vi "Lian_Lab09_II.vi"() -> ()   [LabVIEW 2020]
uses:
  <vilib>/DAQmx/read.llb/DAQmx Read (Analog Wfm 1Chan NSamp).vi
  <vilib>/DAQmx/create/channels.llb/DAQmx Create Channel (AI-Voltage-Basic).vi
  <vilib>/DAQmx/configure/timing.llb/DAQmx Timing (Sample Clock).vi
  <vilib>/measure/macond.llb/IIR Filter for 1 Chan.vi
  <vilib>/measure/maspectr.llb/FFT Spectrum (Mag-Phase) for 1 Chan.vi
  <vilib>/DAQmx/miscellaneous.llb/DAQmx Fill In Error Info.vi
  <vilib>/measure/NI_MAPro.lvlib
  <resource>/objmgr/daqmx.rc
panel:
  out "# Elements \nin Queue":i32
  out "Consumer\nIterations":i32
  out "Producer \nIterations":i32
  out "Actual Rate":dbl
  in  "?":enum32{"Channel", "Sampling", "Filter"}(tab)
  in  "Physical Channels":tag="myDAQ1/ai0"
  in  "Maximum Voltage":dbl=10.0 format="%0.2f"
  in  "Minimum Voltage":dbl=-10.0 format="%0.2f"
  in  "Input Terminal Config.":i32(ring)=10106 items=["Default"=-1, "RSE"=10083, "NRSE"=10078, "Differential"=10106, "Pseudodifferential"=12529]
  in  "Loop Multiple (ms)":u32=1000
  in  "# Samples  per Channel":i32=40000
  in  "Requested Rate":dbl=80000.0 format="%0.2f"
  in  "Samples per Channel":i32=800000
  in  "IIR Specifications":T1={"Topology"=enum."Butterworth", "Type"=enum."Highpass", "Order"=3, "Lower Fc"=100.0, "Upper Fc"=200.0, "PB Ripple"=1.0, "SB Attenuation"=60.0} {"PB Ripple" format="%0.2f"; "SB Attenuation" format="%0.2f"; "Lower Fc" format="%0.2p"; "Upper Fc" format="%0.2p"}
  in  "?":bool
  out "Voltage":waveform(dbl)(graph)
  out "FFT":cluster{"f0":dbl, "df":dbl, "magnitude":dbl[]}(graph)
  # "Settings"
  # "Info"
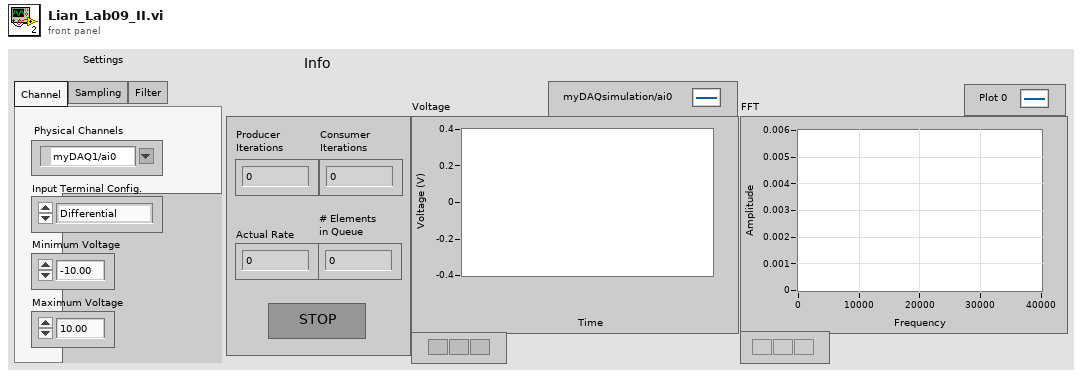
[diagram p1: front panel]
types:
  T1 = cluster{"Topology":enum16{"Off", "Butterworth", "Chebyshev", "Inverse Chebyshev", "Elliptic", "Bessel"}, "Type":enum16{"Lowpass", "Highpass", "Bandpass", "Bandstop"}, "Order":i32, "Lower Fc":dbl, "Upper Fc":dbl, "PB Ripple":dbl, "SB Attenuation":dbl}
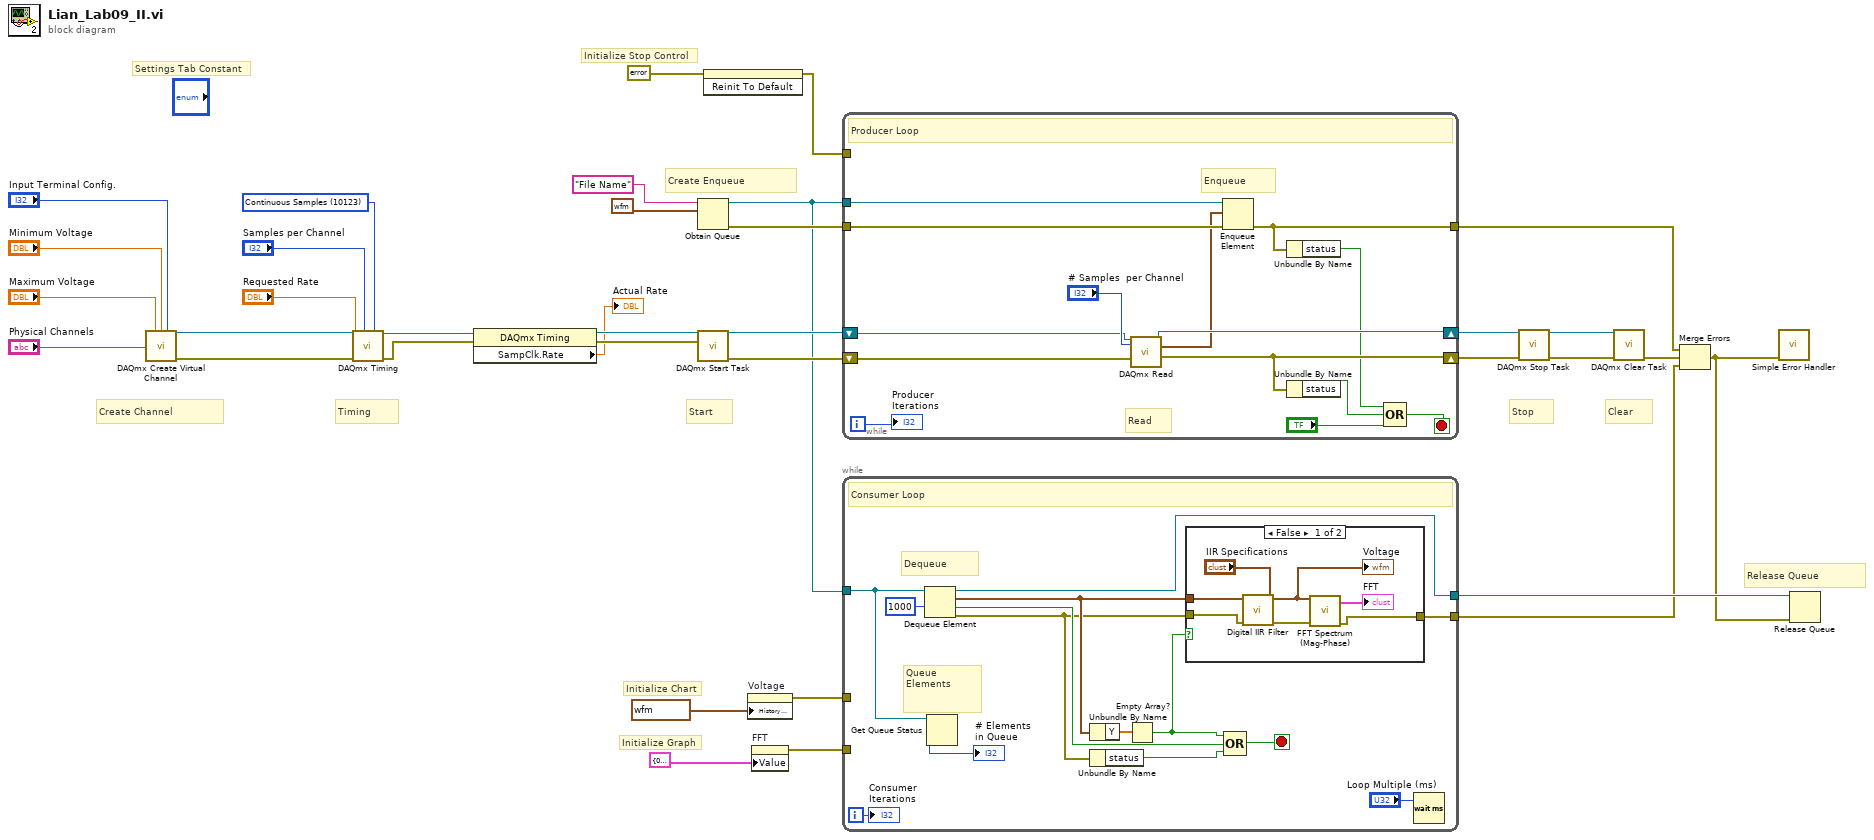
[diagram p0: block diagram]
diagram:
  w21 = 10123 items=["Finite Samples"=10178, "Continuous Samples"=10123, "Hardware Timed Single Point"=12522] ("sample mode")
  # "Initialize Stop Control"
  # "Release Queue"
  # "Create Enqueue"
  # "Clear"
  # "Stop"
  # "Start"
  # "Timing"
  # "Create Channel"
  # "Settings Tab Constant"
  # "Initialize Graph"
  # "Initialize Chart"
  n1 = call-poly <vilib>:"DAQmx Create Virtual Channel.vi"("maximum value"="Maximum Voltage", "minimum value"="Minimum Voltage", "input terminal configuration"="Input Terminal Config.", "physical channels"="Physical Channels") -> ("task out"=w26:refnum<k21>, "error out"=w30:errorcluster)  [unwired: 10 in]
  n2 = call-poly <vilib>:"DAQmx Timing.vi"("task/channels in"=w26, "sample mode"=w21, "samples per channel"="Samples per Channel", "rate"="Requested Rate", "error in"=w30) -> ("task out"=w20:refnum<k21>, "error out"=w18:errorcluster)  [unwired: 9 in]
  n3 = property class="DAQmx Timing"(reference=w20, error in=w18) -> (reference out=w19:refnum<k21>, error out=w17:errorcluster, "SampClk.Rate"=→"Actual Rate":dbl)
  n4 = Obtain Queue(name (unnamed)="File Name", element data type=waveform(dbl) {"t0"=timestamp(0 s since 1904-01-01), "dt"=0.0, "Y"=[]} ("Waveform")) -> (queue out=w12:refnum<queue>, error out=w15:errorcluster)  [unwired: 3 in, 1 out]
  n5 = call <vilib>:"DAQmx Start Task.vi"("task/channels in"=w19, "error in"=w17) -> ("task out"=w25:refnum<k21>, "error out"=w29:errorcluster)  [unwired: 12 in]
  n6 = invoke class="Bool (strict)" method="Reinit To Default"(error in=errorcluster {"status"=FALSE, "code"=0, "source"=""} ("error in (no error)")) -> (error out=w4:errorcluster)  [unwired: 2 in, 2 out]
  n7 = property on="Voltage" class="WFChart (strict)"("History Data"=waveform(dbl)[] [{"t0"=timestamp(0 s since 1904-01-01), "dt"=0.0, "Y"=[]}]) -> (error out=w9:errorcluster)  [unwired: 2 in, 1 out]
  n8 = property on="FFT" class="WFGraph (strict)"("Value"=cluster{"f0":dbl, "df":dbl, "magnitude":dbl[]} {"f0"=0.0, "df"=0.0, "magnitude"=[]} ("FFT")) -> (error out=w10:errorcluster)  [unwired: 2 in, 1 out]
  n9 = while {
    shift-right: [w44] -> w28
    shift-left: w29 -> [w37]
    shift-right: [w49] -> w24
    shift-left: w25 -> [w36]
    tunnel: w12 -> [w48]
    tunnel: w15 -> [w47]
    tunnel: [w45] -> w11
    tunnel: w4 -> [_]
    i -> [w43]
    stop <- w38 stop-if-true
    # "Enqueue"
    # "Read"
    # "Producer Loop"
    n10 = call-poly <vilib>:"DAQmx Read.vi"("task/channels in"=w36, "number of samples per channel"="# Samples  per Channel", "error in"=w37) -> ("task out"=w49:refnum<k21>, "data"=w46:waveform(dbl), "error out"=w44:errorcluster)  [unwired: 10 in]
    n11 = Enqueue Element(queue=w48, element=w46, error in (no error)=w47) -> (error out=w45:errorcluster)  [unwired: 1 in, 2 out]
    n12 = Unbundle By Name(w45) -> ("status"=w39:bool)
    n13 = Unbundle By Name(w44) -> ("status"=w41:bool)
    n14 = Compound Arithmetic op=OR(w39, w41, "?") -> (w38:bool)
    "Producer \nIterations" <- w43
  }
  n15 = while {
    tunnel: w12 -> [w60]
    tunnel: w10 -> [_]
    tunnel: w9 -> [_]
    tunnel: [w54] -> w7
    tunnel: [w50] -> w6
    i -> [w62]
    stop <- w55 stop-if-true
    # "Queue \nElements"
    # "Dequeue"
    # "Consumer Loop"
    n16 = Dequeue Element(queue=w60, timeout in ms (-1)=1000) -> (queue out=w54:refnum<queue>, element=w53:waveform(dbl), timed out?=w57:bool, error out=w51:errorcluster)  [unwired: 1 in]
    n17 = Get Queue Status(queue=w60) -> (# elements in queue=→"# Elements \nin Queue":i32)  [unwired: 2 in, 7 out]
    n18 = Unbundle By Name(w53) -> ("Y"=w59:dbl[])
    n19 = Unbundle By Name(w51) -> ("status"=w58:bool)
    n20 = Empty Array?(array=w59) -> (empty?=w52:bool)
    n21 = case shown="False" w52 {
      tunnel: w53 -> [w68 _]
      tunnel: [w64 w71] -> w50
      tunnel: w51 -> [w66 w71]
      frame False {
        n22 = call-poly <vilib>:"Digital IIR Filter.vi"("IIR filter specifications"="IIR Specifications", "error in (no error)"=w66, "signal in"=w68) -> ("error out"=w65:errorcluster, "signal out"=w67:waveform(dbl))  [unwired: 6 in, 1 out]
        "Voltage" <- w67
        n23 = call-poly <vilib>:"FFT Spectrum (Mag-Phase).vi"("error in (no error)"=w65, "time signal"=w67) -> ("error out"=w64:errorcluster, "magnitude"=→"FFT":cluster{"f0":dbl, "df":dbl, "magnitude":dbl[]})  [unwired: 5 in, 3 out]
      }
      frame True {
      }
    }
    n24 = Compound Arithmetic op=OR(w52, w57, w58) -> (w55:bool)
    n25 = Wait (ms)(milliseconds to wait="Loop Multiple (ms)") -> ()  [unwired: 1 out]
    "Consumer\nIterations" <- w62
  }
  n26 = call <vilib>:"DAQmx Stop Task.vi"("task/channels in"=w24, "error in"=w28) -> ("task out"=w23:refnum<k21>, "error out"=w27:errorcluster)  [unwired: 12 in]
  n27 = call <vilib>:"DAQmx Clear Task.vi"("task in"=w23, "error in"=w27) -> ("error out"=w13:errorcluster)  [unwired: 13 in]
  n28 = Merge Errors(w11, w13, w6) -> (w5:errorcluster)
  n29 = call <vilib>:"Simple Error Handler.vi"("error in (no error)"=w5) -> ()  [unwired: 4 in, 5 out]
  n30 = Release Queue(queue=w7, error in (no error)=w5) -> ()  [unwired: 1 in, 3 out]
